vi "Output Subset.vi"(8 "error in (no error)":errorcluster, 10 "Output subset length":i32, 11 "Spectrum Recorder too in":refnum<class "RP Transceiver.lvclass">) -> (0 "error out":errorcluster, 2 "Output subset":i32[](array[numeric]), 3 "Spectrum Recorder too out":refnum<class "RP Transceiver.lvclass">)   [LabVIEW 2024, in "RP Transceiver.lvclass"]
uses:
  RP Transceiver.lvclass
  RP Transceiver.lvclass/RP Transceiver.ctl
panel:
  out "x > y?":bool
  out "head  length":i32
  out "tail length":i32
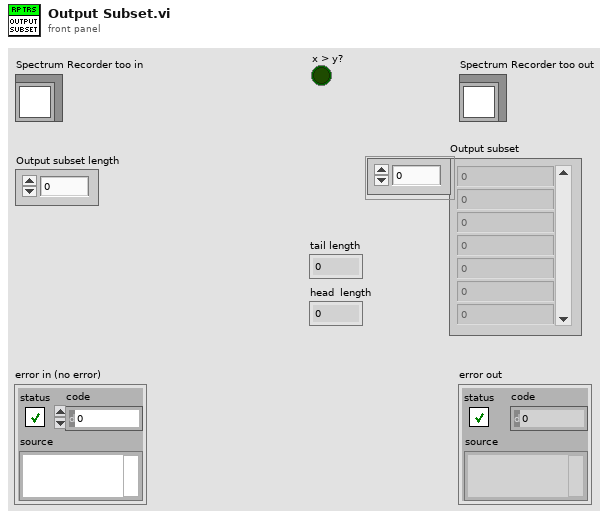
[diagram p1: front panel]
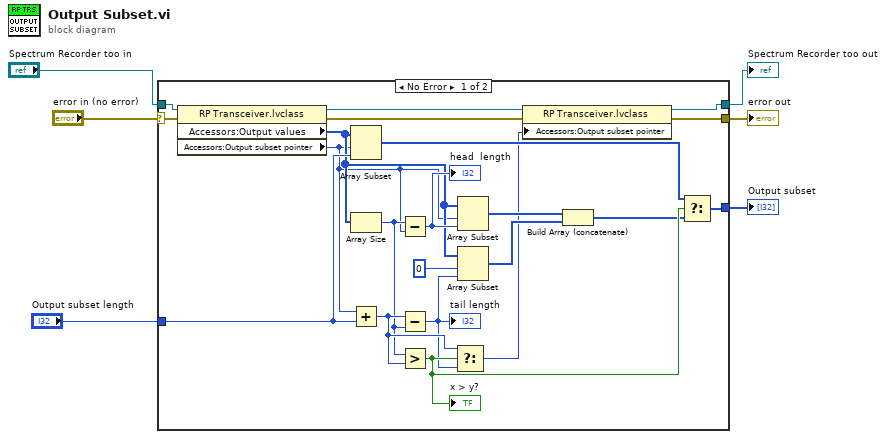
[diagram p0: block diagram]
diagram:
  n1 = case shown="No Error" "error in (no error)" {
    selector: "error in (no error)" -> [w27 w29]
    tunnel: [w10 w29] -> w5
    tunnel: [w9 w28] -> w3
    tunnel: "Spectrum Recorder too in" -> [w14 w28]
    tunnel: "Output subset length" -> [w25 _]
    tunnel: [w7 _] -> w1
    frame No Error {
      n2 = property class="RP Transceiver.lvclass"(reference=w14, error in=w27) -> (reference out=w13:refnum<class "RP Transceiver.lvclass">, error out=w15:errorcluster, "Accessors:Output values"=w12:i32[], "Accessors:Output subset pointer"=w11:i32)
      n3 = Array Subset(array=w12, index=w11, length=w25) -> (w23:i32[])
      n4 = Array Size(array=w12) -> (size(s)=w22:i32)
      n5 = Add(x=w11, y=w25) -> (x+y=w26:i32)
      n6 = Subtract(x=w22, y=w11) -> (x-y=w21:i32)
      "head  length" <- w21
      n7 = Subtract(x=w26, y=w22) -> (x-y=w16:i32)
      "tail length" <- w16
      n8 = Greater?(x=w22, y=w26) -> (0:w24:bool)
      "x > y?" <- w24
      n9 = Select(t=w26, s=w24, f=w16) -> (s? t:f=w8:i32)
      n10 = Array Subset(array=w12, index=w11, length=w21) -> (w19:i32[])
      n11 = Array Subset(array=w12, index=0, length=w16) -> (w18:i32[])
      n12 = property class="RP Transceiver.lvclass"(reference=w13, error in=w15, "Accessors:Output subset pointer"=w8) -> (reference out=w9:refnum<class "RP Transceiver.lvclass">, error out=w10:errorcluster)
      n13 = Build Array (concatenate)(w19, w18) -> (w17:i32[])
      n14 = Select(t=w23, s=w24, f=w17) -> (s? t:f=w7:i32[])
    }
    frame Error {
    }
  }
  "error out" <- w5
  "Spectrum Recorder too out" <- w3
  "Output subset" <- w1
